vi "Launch Database.vi"(0 "Hotel Management Tool Model in":refnum<class "Hotel Management Tool Model.lvclass">, 11 "error in (no error)":errorcluster) -> (4 "Hotel Management Tool Model out":refnum<class "Hotel Management Tool Model.lvclass">, 15 "error out":errorcluster)   [LabVIEW 2023, in "Hotel Management Tool Model.lvlib" / "Hotel Management Tool Model.lvclass"]
uses:
  Hotel Management Tool Model.lvclass
  Hotel Management Tool Model.lvclass/Hotel Management Tool Model.ctl
  File Data Manager/File Data Manager/File Data Manager.lvclass
  Database Data Manager/Database Data Manager/Database Data Manager.lvclass
  <vilib>/ActorFramework/Actor/Actor.lvclass
  C:/Users/bhaghyaraj/Trainings/NI Actor Frameowork/SDLC/Central Data Manager/Central Data Manager/Central Data Manager.lvclass
  C:/Users/bhaghyaraj/Trainings/NI Actor Frameowork/SDLC/Model Base/Model Base/Model Base.lvclass
  C:/Program Files/National Instruments/LabVIEW 2023/vi.lib/ActorFramework/Actor/Actor.lvclass
  C:/Users/bhaghyaraj/Trainings/NI Actor Frameowork/SDLC/Interfaces/Model Base/Incoming Model Base Interface.lvclass
  C:/Users/bhaghyaraj/Trainings/NI Actor Frameowork/SDLC/File Data Manager/File Data Manager/File Data Manager.lvclass
  C:/Users/bhaghyaraj/Trainings/NI Actor Frameowork/SDLC/Database Data Manager/Database Data Manager/Database Data Manager.lvclass
  Central Data Manager/Central Data Manager/Central Data Manager.lvclass
  C:/Users/bhaghyaraj/Trainings/NI Actor Frameowork/SDLC/Hotel Management Tool Model/Hotel Management Tool Model/Hotel Management Tool Model.lvclass
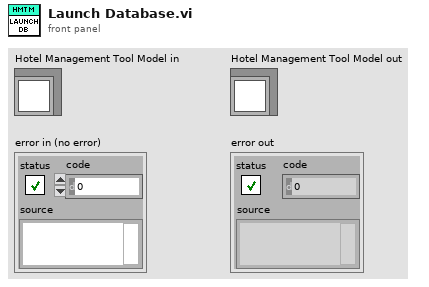
[diagram p1: front panel]
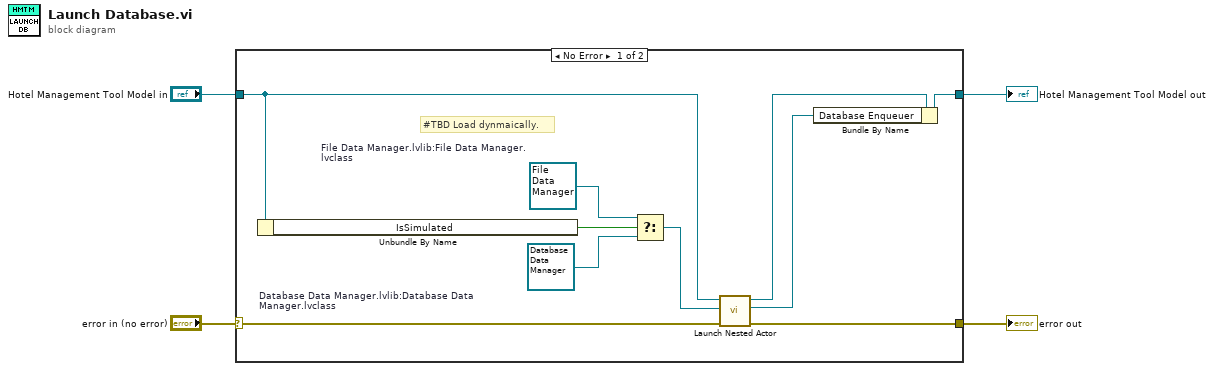
[diagram p0: block diagram]
diagram:
  n1 = case shown="No Error" "error in (no error)" {
    selector: "error in (no error)" -> [w14 w16]
    tunnel: [w10 w16] -> w3
    tunnel: [w7 w15] -> w1
    tunnel: "Hotel Management Tool Model in" -> [w9 w15]
    frame No Error {
      w12 = refnum<class "Database Data Manager.lvclass"> refnum  # Database Data Manager.lvlib:Database Data Manager.lvclass
      w13 = refnum<class "File Data Manager.lvclass"> refnum  # File Data Manager.lvlib:File Data Manager.lvclass
      # "#TBD Load dynmaically."
      n2 = Unbundle By Name(w9) -> ("IsSimulated"=w11:bool)
      n3 = Select(t=w13, s=w11, f=w12) -> (s? t:f=w5:refnum<class "Central Data Manager.lvclass">)
      n4 = call <vilib>:"Launch Nested Actor.vi"("error in (no error)"=w14, "Nested Actor"=w5, "Caller Actor in"=w9) -> ("error out"=w10:errorcluster, "Nested Actor's Enqueuer"=w6:refnum<class "Message Enqueuer.lvclass">, "Caller Actor in"=w8:refnum<class "Hotel Management Tool Model.lvclass">)  [unwired: 6 in]
      n5 = Bundle By Name(cluster=w8, "Database Enqueuer"=w6) -> (w7:refnum<class "Hotel Management Tool Model.lvclass">)
    }
    frame Error {
    }
  }
  "error out" <- w3
  "Hotel Management Tool Model out" <- w1
